vi "querey dcs spot.vi"(0 "Enable":bool=TRUE, 5 "error in (no error)":errorcluster) -> (14 "Spot":T1, 15 "Cancel loading":bool caption="Cancel", 18 "OK":bool, 19 "error out":errorcluster)   [LabVIEW 2013]
doc: "Displays a standard dialog box that prompts users to enter information, such as a user name and password.\n--------------------\n\nThis Express VI is configured as follows:\n\nMessage to Display to the User:\nThe inputs are: \nNumber: Upper Timestamp Range\nNumber: Lower Timestamp Range\nNumber: Settings ID"
uses:
  DCSConstraints.ctl
  <vilib>/Math Plots/3D Math Plots/3D Surface/3D Surface XCtrl/3D Surface.xctl
  <vilib>/Math Plots/3D Math Plots/3D Surface/3D Surface Datatype/3D Surface Datatype.lvclass
  dcs_spot.ctl
  Constraints.ctl
panel:
  in  "experiment settings Okay":bool
  in  "experiment settings dropdown":bool
  out "Current Spot Timestamp:":timestamp
  out "Number of matching spots:":dbl
  in  "Current Spot ID:":i64(ring) items=["Any Spot"=-1]
  out "Orange Cursor Position":dbl[](array[numeric]) min=-12.0 max=12.0 step=0.1 format="%.3g"
  out "3D Surface":refnum<class "3D Plot Datatype.lvclass">[](xcontrol)
  in  "Constraints":T2={"Upper Timestamp Range"=timestamp(0 s since 1904-01-01), "Lower Timestamp Range"=timestamp(0 s since 1904-01-01), "Experiment Group:"="", "Experiment Name:"=[0], "name array"=[], "Dust Spot ID"=0.0}
  in  "OK2":bool
  in  "Cancel":bool
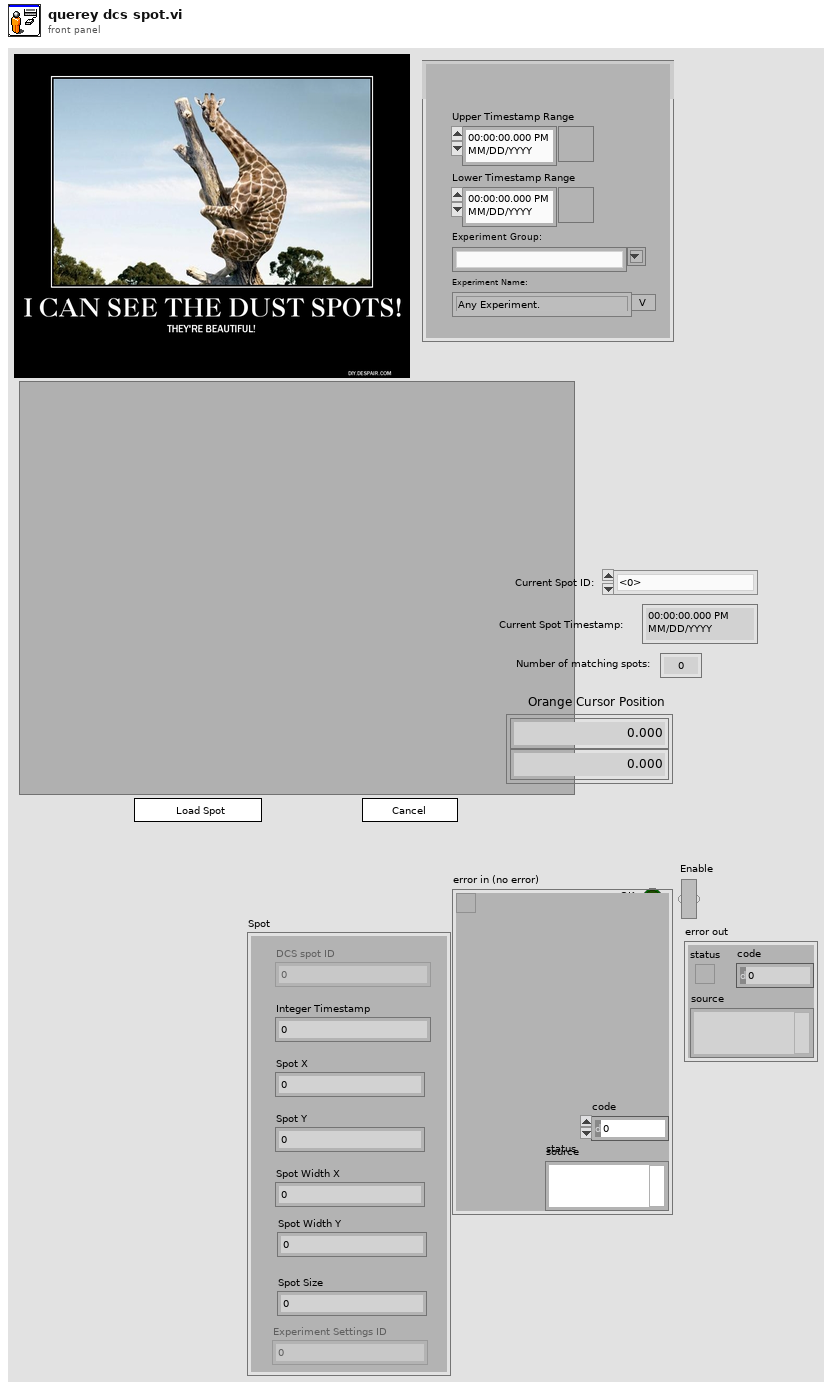
[diagram p1: front panel]
types:
  T1 = typedef "dcs_spot.ctl" = cluster{"DCS spot ID":i32, "Integer Timestamp":i64, "Spot X":dbl, "Spot Y":dbl, "Spot Width X":dbl, "Spot Width Y":dbl, "Spot Size":i32, "Experiment Settings ID":i32}
  T2 = typedef "DCSConstraints.ctl" = cluster{"Upper Timestamp Range":timestamp, "Lower Timestamp Range":timestamp, "Experiment Group:":string, "Experiment Name:":i32[], "name array":string[], "Dust Spot ID":dbl}
  T3 = typedef "Constraints.ctl" = cluster{"Upper Timestamp Range":timestamp, "Lower Timestamp Range":timestamp, "Experiment Group:":string, "Experiment Name:":i32[], "Upper Velocity Limit (km/s)":dbl, "Lower Velocity Limit (km/s)":dbl, "Upper Mass Limit (kg)":dbl, "Lower Mass Limit (kg)":dbl, "name array":string[], "Estimate Quality":cluster{dbl, dbl}}
  T4 = typedef "3D Plot.lvclass/Cursor Property Array.ctl" = T5[]
  T5 = typedef "3D Plot.lvclass/Cursor Property.ctl" = cluster{"Cursor Visible":bool, "Cursor Enable":bool, "Cursor Position":T6, "Cursor Point":T7, "Cursor Line":T9, "Cursor Plane":T11, "Cursor Text":T12}
  T6 = typedef "3D Plot.lvclass/Cursor Position.ctl" = cluster{"Cursor Plot ID":i32, "Cursor X":sgl, "Cursor Y":sgl, "Cursor Z":sgl, "Cursor Snap To":enum16{"Fixed", "Nearest Plot", "Snap to Plot"}}
  T7 = typedef "3D Plot.lvclass/Cursor Point.ctl" = cluster{"Cursor Point Color":u32, "Cursor Point Size":sgl, "Cursor Point Style":T8}
  T8 = typedef "3D Plot.lvclass/Sprite Type.ctl" = enum16{"None", "Empty Square", "Solid Square", "Empty Diamond", "Solid Diamond", "Empty Circle", "Solid Circle", "Asterisk", "Bold X", "Wireframe Sphere", "Solid Sphere", "Wireframe Cube", "Solid Cube"}
  T9 = typedef "3D Plot.lvclass/Cursor Line.ctl" = cluster{"Cursor Line Color":u32, "Cursor Line Width":sgl, "Cursor Line Style":T10}
  T10 = typedef "3D Plot.lvclass/Line Type.ctl" = enum16{"None", "Solid", "Dash", "Dot", "Dash Dot"}
  T11 = typedef "3D Plot.lvclass/Cursor Plane.ctl" = cluster{"Cursor Plane Color":u32, "Cursor Plane Opacity":sgl, "Draw Cursor Plane X-Z":bool, "Draw Cursor Plane Y-Z":bool, "Draw Cursor Plane X-Y":bool}
  T12 = typedef "3D Plot.lvclass/Cursor Text.ctl" = cluster{"Cursor Text":string, "Cursor Text Size":u16, "Cursor Show Position":bool, "Cursor Show Name":bool, "Cursor Text Color":u32, "Background Color":u32, "Background Opacity":sgl}
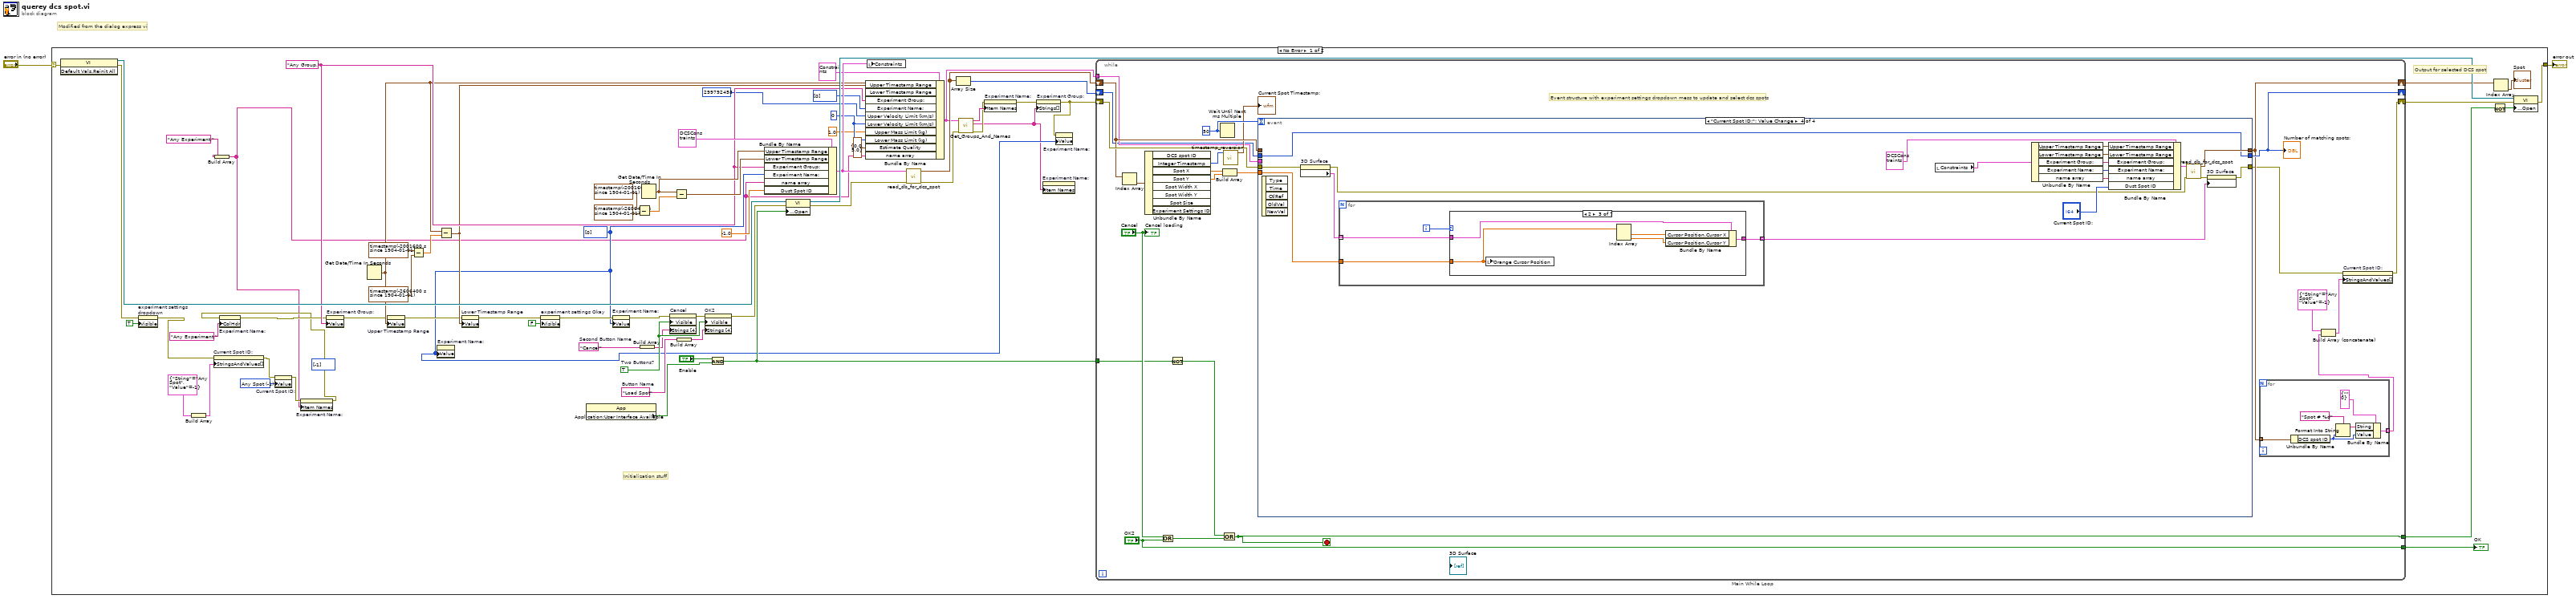
[diagram p0: block diagram]
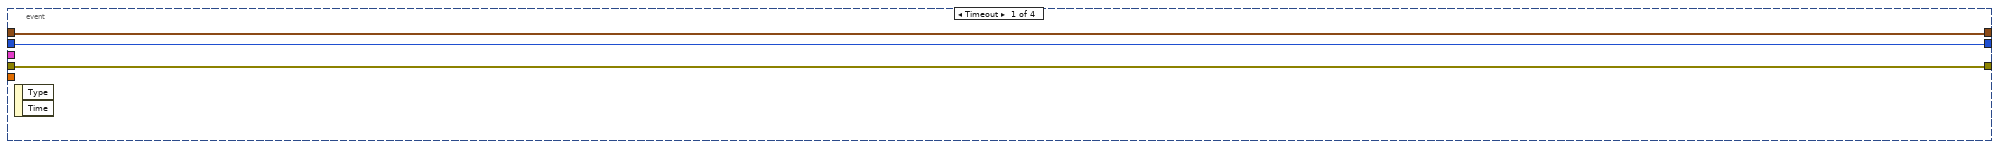
[diagram p2: hidden frame]
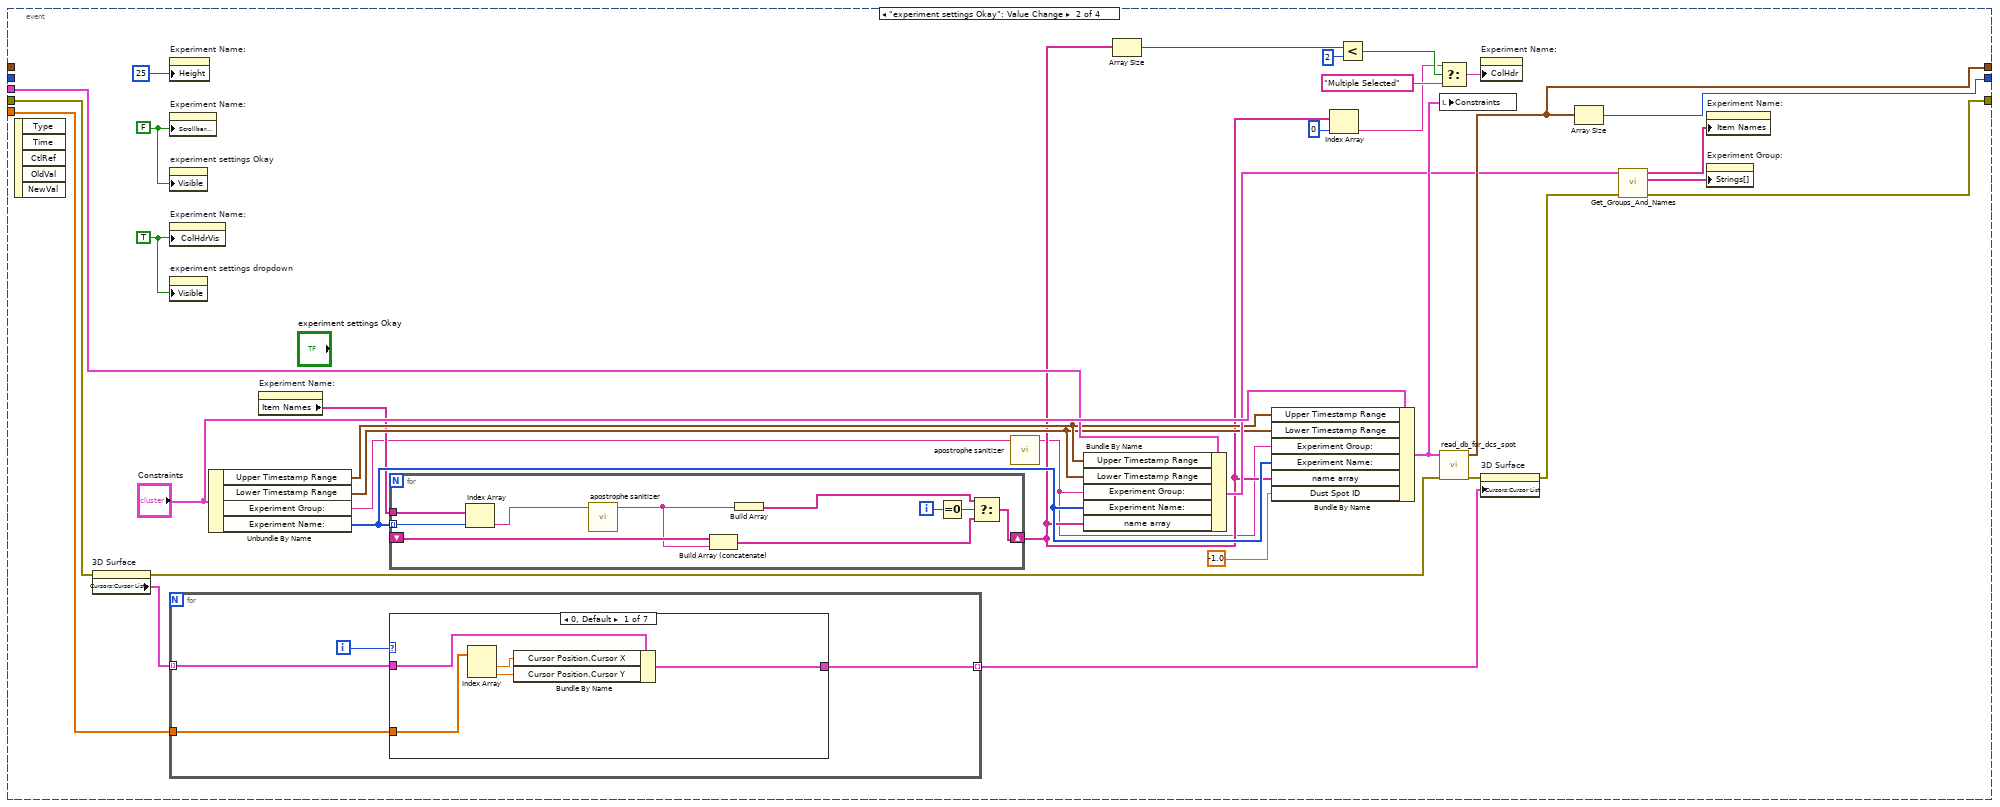
[diagram p3: hidden frame]
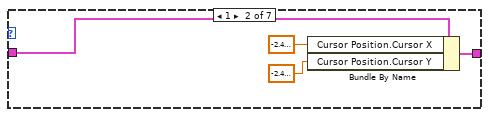
[diagram p4: hidden frame]
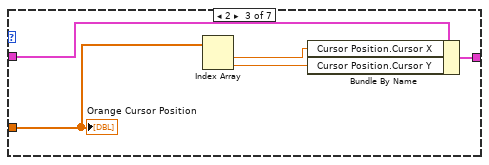
[diagram p5: hidden frame]
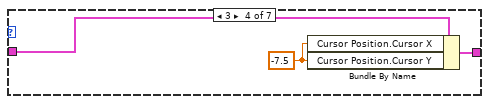
[diagram p6: hidden frame]
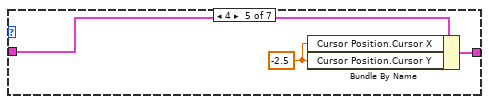
[diagram p7: hidden frame]
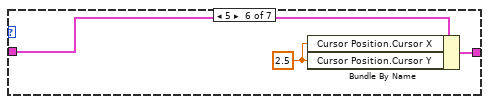
[diagram p8: hidden frame]
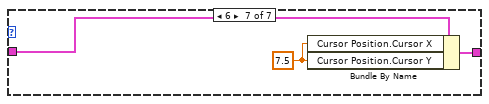
[diagram p9: hidden frame]
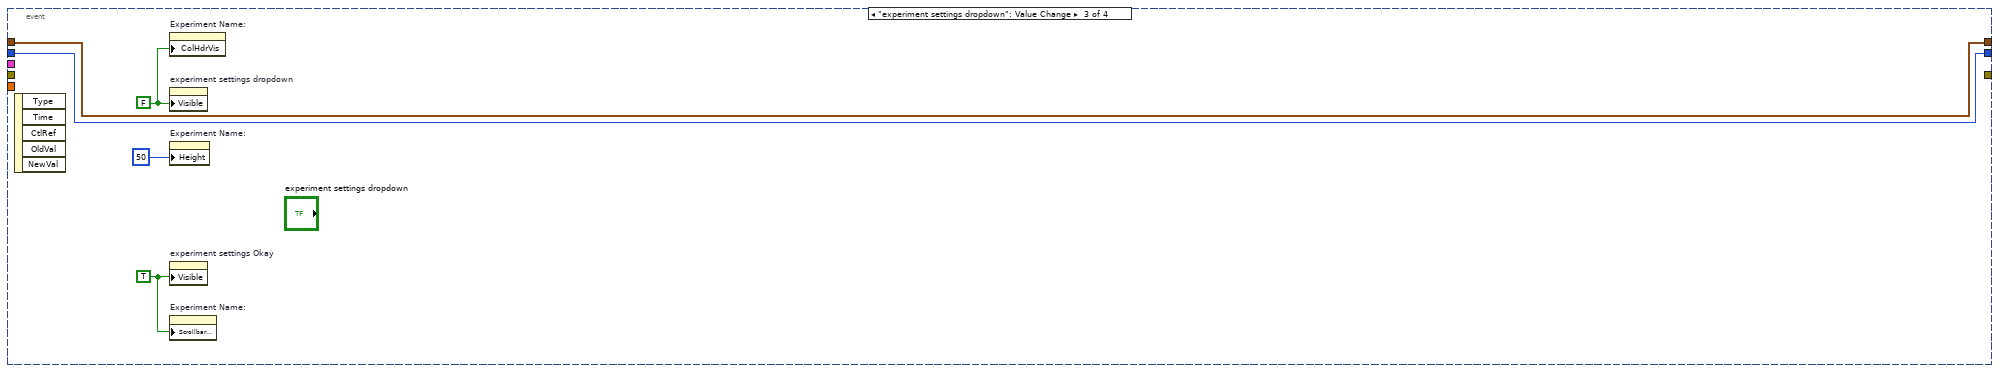
[diagram p10: hidden frame]
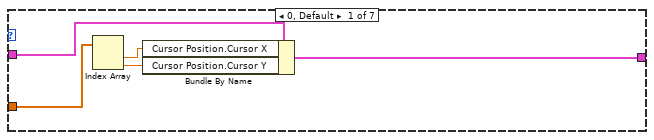
[diagram p11: hidden frame]
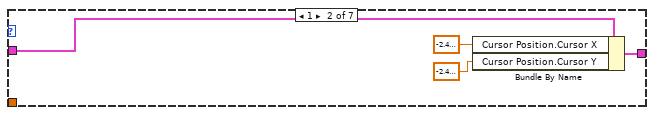
[diagram p12: hidden frame]
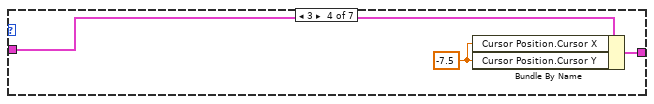
[diagram p13: hidden frame]
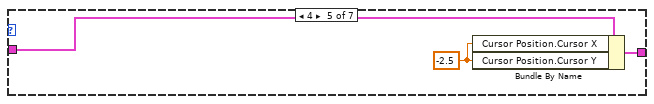
[diagram p14: hidden frame]
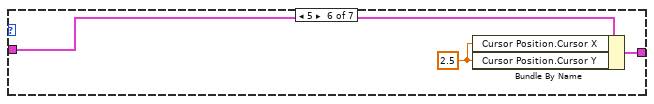
[diagram p15: hidden frame]
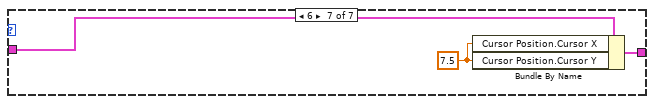
[diagram p16: hidden frame]
diagram:
  # "Modified from the dialog express vi"
  n1 = case shown="No Error" "error in (no error)" {
    selector: "error in (no error)" -> [w25 w233]
    tunnel: [w62 w233] -> w2
    frame No Error {
      (unwired) i32[] [-1] ("Value")
      w13 = i64 -1 items=["Any Spot"=-1, "Spot # 232"=232, "Spot # 233"=233, "Spot # 234"=234, "Spot # 235"=235, "Spot # 236"=236, "Spot # 237"=237, "Spot # 238"=238, "Spot # 239"=239, "Spot # 240"=240] ("Current Spot ID:")
      w38 = i64 0 ("Lower Timestamp Limit")
      w36 = "Any Group." ("element")
      w10 = i32[] [0] ("Experiment Name:")
      w66 = "Cancel"  # Second Button Name
      w64 = "Load Spot"  # Button Name
      w72 = TRUE  # Two Buttons?
      # "Output for selected DCS spot"
      # "Initialization stuff"
      n2 = invoke class="VI" method="Default Vals.Reinit All"(error in=w25) -> (reference out=w59:refnum<vi>, error out=w24:errorcluster)  [unwired: 2 in, 1 out]
      n3 = property on="experiment settings dropdown" class="Bool (strict)"(error in=w24, "Visible"=TRUE) -> (error out=w14:errorcluster)  [unwired: 1 in, 1 out]
      n4 = Build Array(cluster{"String":string, "Value":i64} {"String"="Any Spot", "Value"=-1} ("element")) -> (w15:cluster{"String":string, "Value":i64}[])
      n5 = property on="Current Spot ID:" class="Ring (strict)"(error in=w14, "StringsAndValues[]"=w15) -> (error out=w12:errorcluster)  [unwired: 1 in, 1 out]
      n6 = Build Array("Any Experiment." ("element")) -> (w4:string[])
      n7 = property on="Current Spot ID:" class="Ring (strict)"(error in=w12, "Value"=w13) -> (error out=w7:errorcluster)  [unwired: 1 in, 1 out]
      n8 = property on="Experiment Name:" class="LstBox (strict)"(error in=w7, "Item Names"=w4) -> (error out=w6:errorcluster)  [unwired: 1 in, 1 out]
      n9 = property on="Experiment Name:" class="LstBox (strict)"(error in=w6, "ColHdr"="Any Experiment." ("element")) -> (error out=w8:errorcluster)  [unwired: 1 in, 1 out]
      n10 = property on="Experiment Group:" class="CmbBox"(error in=w8, "Value"=w36) -> (error out=w23:errorcluster)  [unwired: 1 in, 1 out]
      n11 = Get Date/Time In Seconds() -> (seconds since 1Jan1904=w30:timestamp)
      n12 = property on="Upper Timestamp Range" class="AbsTime (strict)"(error in=w23, "Value"=w30) -> (error out=w22:errorcluster)  [unwired: 1 in, 1 out]
      n13 = Subtract(x=timestamp(-2001600 s since 1904-01-01) ("current time"), y=timestamp(-2606400 s since 1904-01-01) ("current time")) -> (x-y=w40:dbl)
      n14 = property on="Experiment Name:" class="LstBox (strict)"("Value"=w10) -> ()  [unwired: 2 in, 2 out]
      n15 = Subtract(x=w30, y=w40) -> (x-y=w29:timestamp)
      n16 = property on="Lower Timestamp Range" class="AbsTime (strict)"(error in=w22, "Value"=w29) -> (error out=w20:errorcluster)  [unwired: 1 in, 1 out]
      n17 = property on="experiment settings Okay" class="Bool (strict)"(error in=w20, "Visible"=FALSE) -> (error out=w19:errorcluster)  [unwired: 1 in, 1 out]
      n18 = property class="App"() -> ("Application:User Interface Available"=w60:bool)  [unwired: 2 in, 2 out]
      n19 = property on="Experiment Name:" class="LstBox (strict)"(error in=w19, "Value"=w10) -> (error out=w21:errorcluster)  [unwired: 1 in, 1 out]
      n20 = Subtract(x=timestamp(-2001600 s since 1904-01-01) ("Lower Timestamp Range"), y=timestamp(-2606400 s since 1904-01-01) ("Lower Timestamp Range")) -> (x-y=w55:dbl)
      n21 = Build Array(w66) -> (w67:string[])
      n22 = Get Date/Time In Seconds() -> (seconds since 1Jan1904=w51:timestamp)
      n23 = property on="Cancel" class="Bool"(error in=w21, "Visible"=w72, "Strings [4]"=w67) -> (error out=w70:errorcluster)  [unwired: 1 in, 1 out]
      n24 = Subtract(x=w51, y=w55) -> (x-y=w50:timestamp)
      n25 = Build Array(w64) -> (w65:string[])
      n26 = property on="OK2" class="Bool"(error in=w70, "Visible"=w72, "Strings [4]"=w65) -> (error out=w58:errorcluster)  [unwired: 1 in, 1 out]
      n27 = And(x="Enable", y=w60) -> (x .and. y?=w54:bool)
      n28 = Bundle By Name(cluster=T2 {"Upper Timestamp Range"=timestamp(0 s since 1904-01-01), "Lower Timestamp Range"=timestamp(0 s since 1904-01-01), "Experiment Group:"="", "Experiment Name:"=[], "name array"=[], "Dust Spot ID"=0.0} ("Constraints"), "Upper Timestamp Range"=w51, "Lower Timestamp Range"=w50, "Experiment Group:"=w36, "Experiment Name:"=w10, "name array"=w4, "Dust Spot ID"=-1.0) -> (w49:T2)
      n29 = property class="VI"(reference=w59, error in=w58, "Front Panel Window:Open"=w54) -> (reference out=w53:refnum<vi>, error out=w47:errorcluster)
      n30 = Bundle By Name(cluster=T3 {"Upper Timestamp Range"=timestamp(0 s since 1904-01-01), "Lower Timestamp Range"=timestamp(0 s since 1904-01-01), "Experiment Group:"="", "Experiment Name:"=[], "Upper Velocity Limit (km/s)"=0.0, "Lower Velocity Limit (km/s)"=0.0, "Upper Mass Limit (kg)"=0.0, "Lower Mass Limit (kg)"=0.0, "name array"=[], "Estimate Quality"={0.0, 0.0}} ("Constraints"), "Upper Timestamp Range"=w30, "Lower Timestamp Range"=w29, "Experiment Group:"=w36, "Experiment Name:"=i32[] [0], "Upper Velocity Limit (km/s)"=299792458, "Lower Velocity Limit (km/s)"=w38, "Upper Mass Limit (kg)"=1.0, "Lower Mass Limit (kg)"=w38, "Estimate Quality"=cluster{dbl, dbl} {0.0, 5.0}, "name array"=w4) -> (w31:T3)
      n31 = local write "Constraints"(w49) -> ()
      n32 = call "read_db_for_dcs_spot.vi"("error in (no error)"=w47, "Constraints"=w49) -> ("error out"=w32:errorcluster, "Array"=w46:T1[])  [unwired: 8 in]
      n33 = Array Size(array=w46) -> (size(s)=w45:i32)
      n34 = call "Get_Groups_And_Names.vi"("error in (no error)"=w32, "Constraints"=w31) -> ("error out"=w18:errorcluster, "Groups"=w9:string[], "Names"=w33:string[])  [unwired: 2 in, 5 out]
      n35 = property on="Experiment Name:" class="LstBox (strict)"(error in=w18, "Item Names"=w33) -> (error out=w17:errorcluster)  [unwired: 1 in, 1 out]
      n36 = property on="Experiment Group:" class="CmbBox"(error in=w17, "Strings[]"=w9) -> (error out=w11:errorcluster)  [unwired: 1 in, 1 out]
      n37 = property on="Experiment Name:" class="LstBox (strict)"("Item Names"=w9) -> ()  [unwired: 2 in, 2 out]
      n38 = property on="Experiment Name:" class="LstBox (strict)"(error in=w11, "Value"=w10) -> ()  [unwired: 1 in, 2 out]
      n39 = while "Main While Loop" {
        tunnel: ["OK2"] -> w71
        tunnel: w54 -> [w95]
        tunnel: [w93] -> w68
        shift-right: [w76] -> w63
        shift-left: w11 -> [w90]
        shift-right: [w80] -> _
        shift-left: w45 -> [w79]
        shift-right: [w78] -> w44
        shift-left: w46 -> [w87]
        tunnel: w31 -> [w81]
        stop <- w93 stop-if-true
        w89 = u32 50 ("millisecond multiple")
        # "Event structure with experiment settings dropdown mess to update and select dcs spots"
        n40 = Index Array(array=w87) -> (element=w88:T1)  [unwired: 1 in]
        n41 = Unbundle By Name(w88) -> ("Integer Timestamp"=w85:i64, "Spot X"=w83:dbl, "Spot Y"=w82:dbl)  [unwired: 5 out]
        n42 = Or(x="Cancel", y="OK2") -> (x .or. y?=w92:bool)
        n43 = Not(x=w95) -> (.not. x?=w94:bool)
        n44 = Wait Until Next ms Multiple(millisecond multiple=w89) -> ()  [unwired: 1 out]
        n45 = Build Array(w83, w82) -> (w84:dbl[])
        n46 = call "timestamp_reversion.vi"("Integer Timestamp"=w85) -> ("time stamp"=→"Current Spot Timestamp:":timestamp)  [unwired: 8 in, 1 out]
        n47 = Compound Arithmetic op=OR(w94, w92) -> (w93:bool)
        n48 = event shown="[3] \"Current Spot ID:\": Value Change" {
          selector: _ -> [_ _ _ _]
          dyn-events: _ -> [_ _ _ _]
          timeout: w89 -> [_ _ _ _]
          tunnel: w90 -> [w105 w137 _ w199]
          tunnel: [w105 w119 _ w200] -> w77
          tunnel: w79 -> [w104 _ w184 w189]
          tunnel: [w104 w136 w184 w189] -> w80
          tunnel: [w103 w132 w183 w190] -> w78
          tunnel: w87 -> [w103 _ w183 _]
          tunnel: w84 -> [_ w129 _ w186]
          tunnel: w81 -> [_ w126 _ _]
          event Timeout {
            n49 = event-data() -> ()  [unwired: 1 in, 2 out]
          }
          event "experiment settings Okay": Value Change {
            w118 = FALSE ("Visible")
            w117 = TRUE ("Visible")
            n50 = event-data() -> ()  [unwired: 1 in, 5 out]
            n51 = property on="3D Surface" class="3D Surface (strict)"(error in=w137) -> (error out=w131:errorcluster, "Cursors:Cursor List"=w138:T4)  [unwired: 1 in, 1 out]
            n52 = property on="Experiment Name:" class="LstBox (strict)"("Height"=u32 25 ("Size:Height")) -> ()  [unwired: 2 in, 2 out]
            n53 = property on="Experiment Name:" class="LstBox (strict)"("Scrollbar Visible"=w118) -> ()  [unwired: 2 in, 2 out]
            n54 = property on="experiment settings Okay" class="Bool (strict)"("Visible"=w118) -> ()  [unwired: 2 in, 2 out]
            n55 = property on="Experiment Name:" class="LstBox (strict)"("ColHdrVis"=w117) -> ()  [unwired: 2 in, 2 out]
            n56 = property on="experiment settings dropdown" class="Bool (strict)"("Visible"=w117) -> ()  [unwired: 2 in, 2 out]
            n57 = for {
              tunnel: w138 -> [w153] mode=indexing
              tunnel: [w151] -> w139 mode=indexing
              tunnel: w129 -> [w150]
              i -> [w152]
              n58 = case shown="0, Default" w152 {
                tunnel: w153 -> [w158 w161 w166 w170 w173 w176 w179]
                tunnel: [w157 w162 w167 w169 w172 w175 w178] -> w151
                tunnel: w150 -> [w156 _ w163 _ _ _ _]
                frame 0, Default {
                  n59 = Index Array(array=w156) -> (element #1=w155:dbl, element #2=w154:dbl)  [unwired: 2 in]
                  n60 = Bundle By Name(cluster=w158, "Cursor Position.Cursor X"=w155, "Cursor Position.Cursor Y"=w154) -> (w157:T5)
                }
                frame 1 {
                  n61 = Bundle By Name(cluster=w161, "Cursor Position.Cursor X"=sgl -2.4, "Cursor Position.Cursor Y"=sgl -2.4) -> (w162:T5)
                }
                frame 2 {
                  n62 = Index Array(array=w163) -> (element #1=w165:dbl, element #2=w164:dbl)  [unwired: 2 in]
                  n63 = Bundle By Name(cluster=w166, "Cursor Position.Cursor X"=w165, "Cursor Position.Cursor Y"=w164) -> (w167:T5)
                  "Orange Cursor Position" <- w163
                }
                frame 3 {
                  w168 = -7.5 ("index")
                  n64 = Bundle By Name(cluster=w170, "Cursor Position.Cursor X"=w168, "Cursor Position.Cursor Y"=w168) -> (w169:T5)
                }
                frame 4 {
                  w171 = -2.5 ("index")
                  n65 = Bundle By Name(cluster=w173, "Cursor Position.Cursor X"=w171, "Cursor Position.Cursor Y"=w171) -> (w172:T5)
                }
                frame 5 {
                  w174 = 2.5 ("index")
                  n66 = Bundle By Name(cluster=w176, "Cursor Position.Cursor X"=w174, "Cursor Position.Cursor Y"=w174) -> (w175:T5)
                }
                frame 6 {
                  w177 = 7.5 ("index")
                  n67 = Bundle By Name(cluster=w179, "Cursor Position.Cursor X"=w177, "Cursor Position.Cursor Y"=w177) -> (w178:T5)
                }
              }
            }
            n68 = Unbundle By Name("Constraints") -> ("Upper Timestamp Range"=w125:timestamp, "Lower Timestamp Range"=w124:timestamp, "Experiment Group:"=w107:string, "Experiment Name:"=w123:i32[])
            n69 = property on="Experiment Name:" class="LstBox (strict)"() -> ("Item Names"=w108:string[])  [unwired: 2 in, 2 out]
            n70 = for {
              tunnel: w123 -> [w148] mode=indexing
              tunnel: w108 -> [w149]
              shift-right: [w142] -> w109
              shift-left: _ -> [w143]
              i -> [w144]
              n71 = Index Array(array=w149, index=w148) -> (element=w141:string)
              n72 = call "apostrophe sanitizer.vi"("imput to db"=w141) -> ("fixed imput to db"=w140:string)  [unwired: 8 in, 2 out]
              n73 = Build Array (concatenate)(w143, w140) -> (w147:string[])
              n74 = Build Array(w140) -> (w146:string[])
              n75 = Equal To 0?(x=w144) -> (x = 0?=w145:bool)
              n76 = Select(t=w146, s=w145, f=w147) -> (s? t:f=w142:string[])
            }
            n77 = call "apostrophe sanitizer.vi"("imput to db"=w107) -> ("fixed imput to db"=w106:string)  [unwired: 8 in, 2 out]
            n78 = Bundle By Name(cluster=w126, "Upper Timestamp Range"=w125, "Lower Timestamp Range"=w124, "Experiment Group:"=w106, "Experiment Name:"=w123, "name array"=w109) -> (w127:T3)
            n79 = Array Size(array=w109) -> (size(s)=w114:i32)
            n80 = Bundle By Name(cluster="Constraints", "Upper Timestamp Range"=w125, "Lower Timestamp Range"=w124, "Experiment Group:"=w106, "Experiment Name:"=w123, "name array"=w109, "Dust Spot ID"=-1.0) -> (w133:T2)
            n81 = Index Array(array=w109, index=0) -> (element=w113:string)
            n82 = Less?(x=w114, y=2) -> (x < y?=w115:bool)
            n83 = Select(t=w113, s=w115, f="Multiple Selected") -> (s? t:f=w112:string)
            n84 = local write "Constraints"(w133) -> ()
            n85 = call "read_db_for_dcs_spot.vi"("error in (no error)"=w131, "Constraints"=w133) -> ("error out"=w130:errorcluster, "Array"=w132:T1[])  [unwired: 8 in]
            n86 = property on="Experiment Name:" class="LstBox (strict)"("ColHdr"=w112) -> ()  [unwired: 2 in, 2 out]
            n87 = property on="3D Surface" class="3D Surface (strict)"(error in=w130, "Cursors:Cursor List"=w139) -> (error out=w120:errorcluster)  [unwired: 1 in, 1 out]
            n88 = Array Size(array=w132) -> (size(s)=w136:i32)
            n89 = call "Get_Groups_And_Names.vi"("error in (no error)"=w120, "Constraints"=w127) -> ("error out"=w119:errorcluster, "Groups"=w121:string[], "Names"=w122:string[])  [unwired: 2 in, 5 out]
            n90 = property on="Experiment Name:" class="LstBox (strict)"("Item Names"=w122) -> ()  [unwired: 2 in, 2 out]
            n91 = property on="Experiment Group:" class="CmbBox"("Strings[]"=w121) -> ()  [unwired: 2 in, 2 out]
          }
          event "experiment settings dropdown": Value Change {
            w180 = TRUE ("Visible Items:Vertical Scrollbar Visible")
            w181 = FALSE ("Visible Items:Vertical Scrollbar Visible")
            n92 = event-data() -> ()  [unwired: 1 in, 5 out]
            n93 = property on="Experiment Name:" class="LstBox (strict)"("ColHdrVis"=w181) -> ()  [unwired: 2 in, 2 out]
            n94 = property on="experiment settings dropdown" class="Bool (strict)"("Visible"=w181) -> ()  [unwired: 2 in, 2 out]
            n95 = property on="Experiment Name:" class="LstBox (strict)"("Height"=50 ("x")) -> ()  [unwired: 2 in, 2 out]
            n96 = property on="experiment settings Okay" class="Bool (strict)"("Visible"=w180) -> ()  [unwired: 2 in, 2 out]
            n97 = property on="Experiment Name:" class="LstBox (strict)"("Scrollbar Visible"=w180) -> ()  [unwired: 2 in, 2 out]
          }
          event "Current Spot ID:": Value Change {
            n98 = event-data() -> ()  [unwired: 1 in, 5 out]
            n99 = property on="3D Surface" class="3D Surface (strict)"(error in=w199) -> (error out=w188:errorcluster, "Cursors:Cursor List"=w201:T4)  [unwired: 1 in, 1 out]
            n100 = for {
              tunnel: w201 -> [w206] mode=indexing
              tunnel: [w204] -> w202 mode=indexing
              tunnel: w186 -> [w203]
              i -> [w205]
              n101 = case shown="2" w205 {
                tunnel: w206 -> [w211 w214 w219 w223 w226 w229 w232]
                tunnel: [w210 w215 w220 w222 w225 w228 w231] -> w204
                tunnel: w203 -> [w209 _ w218 _ _ _ _]
                frame 0, Default {
                  n102 = Index Array(array=w209) -> (element #1=w208:dbl, element #2=w207:dbl)  [unwired: 2 in]
                  n103 = Bundle By Name(cluster=w211, "Cursor Position.Cursor X"=w208, "Cursor Position.Cursor Y"=w207) -> (w210:T5)
                }
                frame 1 {
                  n104 = Bundle By Name(cluster=w214, "Cursor Position.Cursor X"=sgl -2.4, "Cursor Position.Cursor Y"=sgl -2.4) -> (w215:T5)
                }
                frame 2 {
                  n105 = local write "Orange Cursor Position"(w218) -> ()
                  n106 = Index Array(array=w218) -> (element #1=w217:dbl, element #2=w216:dbl)  [unwired: 2 in]
                  n107 = Bundle By Name(cluster=w219, "Cursor Position.Cursor X"=w217, "Cursor Position.Cursor Y"=w216) -> (w220:T5)
                }
                frame 3 {
                  w221 = -7.5 ("index")
                  n108 = Bundle By Name(cluster=w223, "Cursor Position.Cursor X"=w221, "Cursor Position.Cursor Y"=w221) -> (w222:T5)
                }
                frame 4 {
                  w224 = -2.5 ("index")
                  n109 = Bundle By Name(cluster=w226, "Cursor Position.Cursor X"=w224, "Cursor Position.Cursor Y"=w224) -> (w225:T5)
                }
                frame 5 {
                  w227 = 2.5 ("index")
                  n110 = Bundle By Name(cluster=w229, "Cursor Position.Cursor X"=w227, "Cursor Position.Cursor Y"=w227) -> (w228:T5)
                }
                frame 6 {
                  w230 = 7.5 ("index")
                  n111 = Bundle By Name(cluster=w232, "Cursor Position.Cursor X"=w230, "Cursor Position.Cursor Y"=w230) -> (w231:T5)
                }
              }
            }
            n112 = local read "Constraints"() -> (w192:T2)
            n113 = Unbundle By Name(w192) -> ("Upper Timestamp Range"=w194:timestamp, "Lower Timestamp Range"=w195:timestamp, "Experiment Group:"=w196:string, "Experiment Name:"=w198:i32[], "name array"=w197:string[])
            n114 = Bundle By Name(cluster=T2 {"Upper Timestamp Range"=timestamp(0 s since 1904-01-01), "Lower Timestamp Range"=timestamp(0 s since 1904-01-01), "Experiment Group:"="", "Experiment Name:"=[], "name array"=[], "Dust Spot ID"=0.0} ("Constraints"), "Upper Timestamp Range"=w194, "Lower Timestamp Range"=w195, "Experiment Group:"=w196, "Experiment Name:"=w198, "name array"=w197, "Dust Spot ID"="Current Spot ID:") -> (w191:T2)
            n115 = call "read_db_for_dcs_spot.vi"("error in (no error)"=w188, "Constraints"=w191) -> ("error out"=w187:errorcluster, "Array"=w190:T1[])  [unwired: 8 in]
            n116 = property on="3D Surface" class="3D Surface (strict)"(error in=w187, "Cursors:Cursor List"=w202) -> (error out=w200:errorcluster)  [unwired: 1 in, 1 out]
          }
        }
        "Number of matching spots:" <- w80
        n117 = for {
          tunnel: w78 -> [w102] mode=indexing
          tunnel: [w100] -> w74 mode=indexing
          n118 = Unbundle By Name(w102) -> ("DCS spot ID"=w98:i32)
          n119 = Format Into String(format string="Spot # %d", w98) -> (resulting string=w99:string)  [unwired: 2 in, 1 out]
          n120 = Bundle By Name(cluster=cluster{"String":string, "Value":i64} {"String"="", "Value"=0} ("element"), "String"=w99, "Value"=w98) -> (w100:cluster{"String":string, "Value":i64})
        }
        n121 = Build Array (concatenate)(cluster{"String":string, "Value":i64} {"String"="Any Spot", "Value"=-1} ("element"), w74) -> (w75:cluster{"String":string, "Value":i64}[])
        n122 = property on="Current Spot ID:" class="Ring (strict)"(error in=w77, "StringsAndValues[]"=w75) -> (error out=w76:errorcluster)  [unwired: 1 in, 1 out]
        "Cancel loading" <- "Cancel"
      }
      "OK" <- w71
      n123 = Not(x=w68) -> (.not. x?=w69:bool)
      n124 = Index Array(array=w44) -> (element=→"Spot":T1)  [unwired: 1 in]
      n125 = property class="VI"(reference=w53, error in=w63, "Front Panel Window:Open"=w69) -> (error out=w62:errorcluster)  [unwired: 1 out]
    }
    frame Error {
    }
  }
  "error out" <- w2
